vi "Configure.vi"(8 "error in (no error)":errorcluster, 9 "Resolution":enum16{"5 1/2 Digits", "6 1/2 Digits"}(ring), 10 "Range":enum16{"1V", "10V", "100V"}(ring), 11 "DAQ in":refnum<class "DAQ.lvclass">) -> (0 "error out":errorcluster, 3 "DAQ out":refnum<class "DAQ.lvclass">)   [LabVIEW 2024, in "HAL_Example.lvlib" / "DAQ.lvclass"]
uses:
  DAQ.lvclass
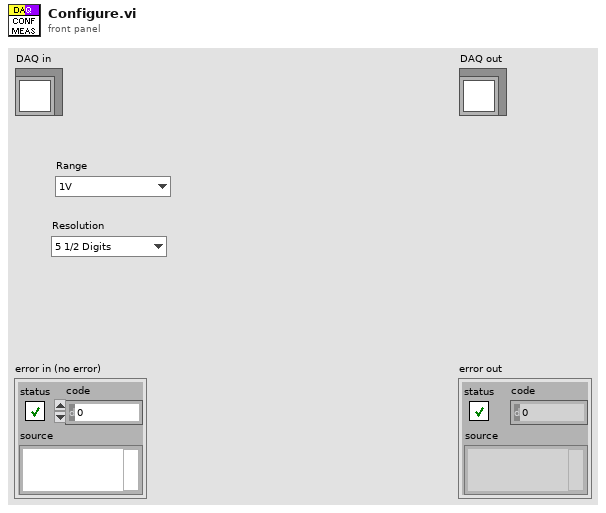
[diagram p1: front panel]
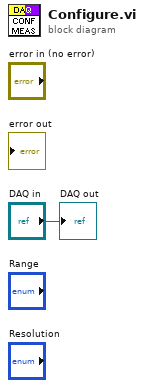
[diagram p0: block diagram]
diagram:
  "DAQ out" <- "DAQ in"
